vi "PM100D_GetRngIndex.vi"(5 "error in (no error)":errorcluster, 11 "VISA in":refnum<visa-resource-name>) -> (0 "error out":errorcluster, 1 "SensType":i32 min=0 max=5, 2 "Rng_Array":string[](array[string]), 3 "dup VISA session":refnum<visa-resource-name>, 4 "IndexOut":i32, 9 "AutoOut":bool)   [LabVIEW 2015]
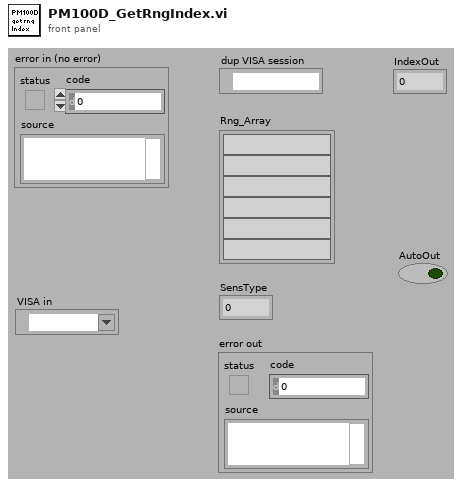
[diagram p1: front panel]
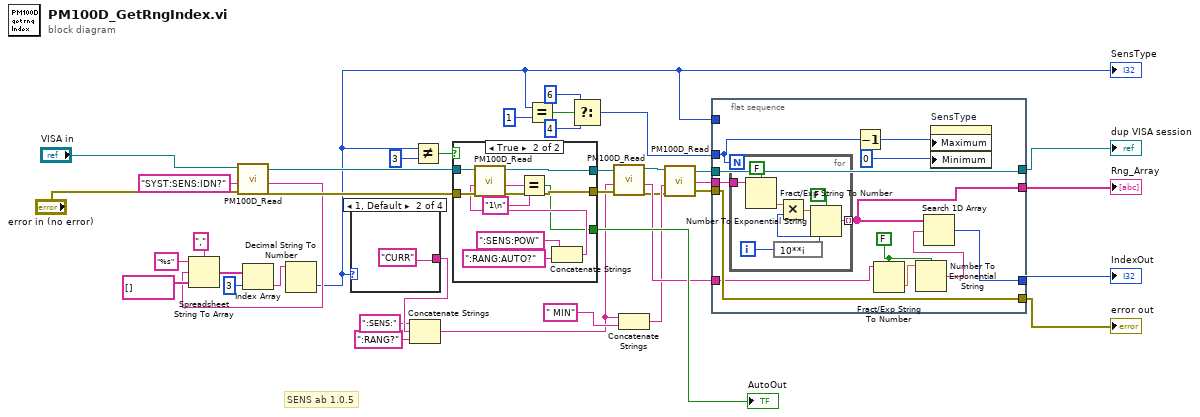
[diagram p0: block diagram]
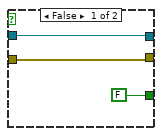
[diagram p2: hidden frame]
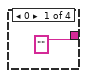
[diagram p3: hidden frame]
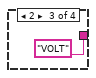
[diagram p4: hidden frame]
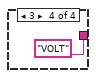
[diagram p5: hidden frame]
diagram:
  # "SENS ab 1.0.5"
  n1 = call "PM100D_Read.vi"("error in (no error)"="error in (no error)", "Command"="SYST:SENS:IDN?", "VISA in"="VISA in") -> ("error out"=w35:errorcluster, "ReadValue"=w26:string, "VISA out"=w33:refnum<visa-resource-name>)  [unwired: 6 in]
  n2 = Spreadsheet String To Array(delimiter (Tab)=",", format string="%s", spreadsheet string=w26, array type (2D Dbl)=string[] [] ("Rng_Array")) -> (array=w28:string[])
  n3 = Index Array(array=w28, index=3) -> (element=w31:string)
  n4 = Decimal String To Number(string=w31) -> (number=w3:i32)  [unwired: 2 in, 1 out]
  "SensType" <- w3
  n5 = case shown="1, Default" w3 {
    tunnel: ["" "CURR" "VOLT" "VOLT"] -> w20
    frame 0 {
    }
    frame 1, Default {
    }
    frame 2 {
    }
    frame 3 {
    }
  }
  n6 = Concatenate Strings(":SENS:" ("string"), w20, ":RANG?" ("string")) -> (w8:string)
  n7 = Not Equal?(x=w3, y=3) -> (x != y?=w38:bool)
  n8 = case shown="True" w38 {
    tunnel: w33 -> [w46 w56]
    tunnel: [w46 w55] -> w34
    tunnel: w35 -> [w45 w54]
    tunnel: [w45 w53] -> w36
    tunnel: [FALSE w47] -> w39
    frame False {
    }
    frame True {
      n9 = Concatenate Strings(":SENS:POW" ("string"), ":RANG:AUTO?" ("string")) -> (w52:string)
      n10 = call "PM100D_Read.vi"("error in (no error)"=w54, "Command"=w52, "VISA in"=w56) -> ("error out"=w53:errorcluster, "ReadValue"=w49:string, "VISA out"=w55:refnum<visa-resource-name>)  [unwired: 6 in]
      n11 = Equal?(x=w49, y="1\n") -> (x = y?=w47:bool)
    }
  }
  "AutoOut" <- w39
  n12 = Equal?(x=w3, y=1) -> (x = y?=w22:bool)
  n13 = Select(t=6, s=w22, f=4) -> (s? t:f=w11:i32)
  n14 = call "PM100D_Read.vi"("error in (no error)"=w36, "Command"=w8, "VISA in"=w34) -> ("error out"=w6:errorcluster, "ReadValue"=w17:string, "VISA out"=w5:refnum<visa-resource-name>)  [unwired: 6 in]
  n15 = Concatenate Strings(w8, " MIN" ("string")) -> (w9:string)
  n16 = call "PM100D_Read.vi"("error in (no error)"=w6, "Command"=w9, "VISA in"=w5) -> ("error out"=w15:errorcluster, "ReadValue"=w16:string, "VISA out"=w14:refnum<visa-resource-name>)  [unwired: 6 in]
  n17 = flat-sequence {
    tunnel: w11 -> [w60]
    tunnel: w14 -> [w68]
    tunnel: [w68] -> w18
    tunnel: [w67] -> w19
    tunnel: w15 -> [w67]
    tunnel: w16 -> [w66]
    tunnel: w17 -> [w65]
    tunnel: [w61] -> w4
    tunnel: [w59] -> w2
    tunnel: w3 -> [_]
    frame #0 {
      w63 = FALSE ("use system decimal point (T)")
      n18 = for {
        N: w60 -> [_]
        tunnel: w66 -> [w75]
        tunnel: [w69] -> w61 mode=indexing
        i -> [w76]
        n19 = Fract/Exp String To Number(use system decimal point (T)=FALSE, string=w75) -> (number=w74:dbl)  [unwired: 2 in, 1 out]
        n20 = expression code="10**i"(w76) -> (w73:i32)
        n21 = Multiply(x=w74, y=w73) -> (x*y=w71:dbl)
        n22 = Number To Exponential String(number=w71, 1:FALSE ("use system decimal point (T)")) -> (E-format string=w69:string)  [unwired: 2 in]
      }
      n23 = Decrement(x=w60) -> (x-1=w58:i32)
      n24 = Fract/Exp String To Number(use system decimal point (T)=w63, string=w65) -> (number=w64:dbl)  [unwired: 2 in, 1 out]
      n25 = Number To Exponential String(number=w64, 1:w63) -> (E-format string=w62:string)  [unwired: 2 in]
      n26 = Search 1D Array(1D array=w61, element=w62) -> (index of element=w59:i32)  [unwired: 1 in]
      n27 = property on="SensType" class="DigNum (strict)"("Maximum"=w58, "Minimum"=0) -> ()  [unwired: 2 in, 2 out]
    }
  }
  "Rng_Array" <- w4
  "error out" <- w19
  "dup VISA session" <- w18
  "IndexOut" <- w2
